vi "图片处理2.vi"() -> ()   [LabVIEW 2018]
uses:
  <vilib>/userdefined/High Color/IMAQdx.ctl
  <vilib>/vision/NI_Vision_Development_Module.lvlib
  <vilib>/vision/driver/NI_Vision_Acquisition_Software.lvlib
panel:
  out "Image 2":T1(plugin-control)
  out "Image":T1(plugin-control)
  in  "File Path":path
  in  "停止":bool
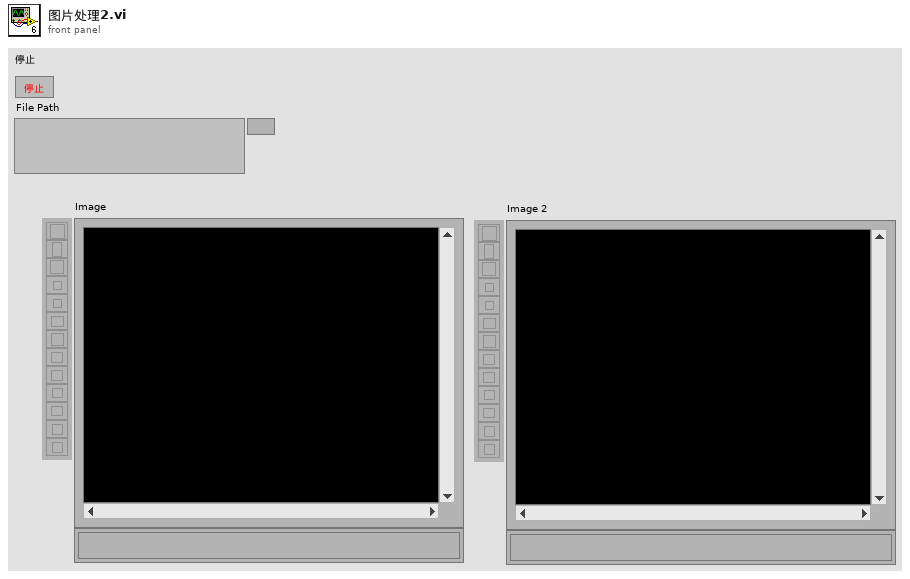
[diagram p1: front panel]
types:
  T1 = typedef "IMAQ Image.ctl" = refnum<image>
  T2 = typedef "IMAQdx.ctl" = refnum<k21>
  T3 = cluster{"Position":cluster{"x":sgl, "y":sgl}, "Angle":sgl, "Scale":sgl, "Score":sgl, "Bounding Box":cluster{"x":sgl, "y":sgl}[]}[]
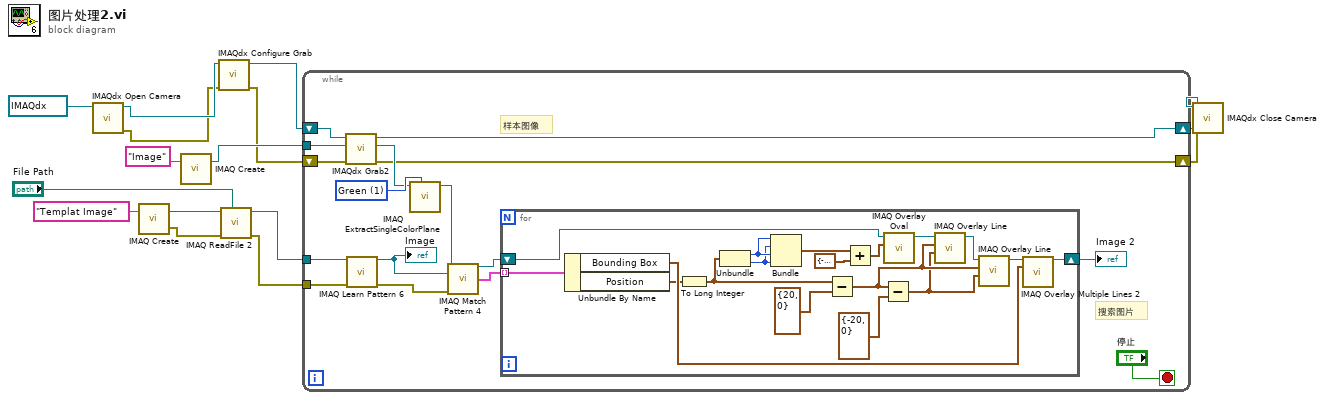
[diagram p0: block diagram]
diagram:
  n1 = call <vilib>:"IMAQdx Open Camera.vi"("Session In"=T2 "cam0") -> ("error out"=w3:errorcluster, "Session Out"=w4:T2)  [unwired: 9 in]
  n2 = call "IMAQ Create"("Image Name"="Templat Image") -> ("New Image"=w15:T1, "error out"=w13:errorcluster)  [unwired: 4 in]
  n3 = call "IMAQ Create"("Image Name"="Image") -> ("New Image"=w10:T1)  [unwired: 4 in, 1 out]
  n4 = call <vilib>:"IMAQdx Configure Grab.vi"("error in"=w3, "Session In"=w4) -> ("error out"=w1:errorcluster, "Session Out"=w2:T2)  [unwired: 8 in]
  n5 = call "IMAQ ReadFile 2"("File Path"="File Path", "error in (no error)"=w13, "Image"=w15) -> ("error out"=w12:errorcluster, "Image Out"=w14:T1)  [unwired: 4 in, 3 out]
  n6 = while {
    tunnel: w14 -> [w31]
    tunnel: w12 -> [w30]
    shift-right: [w17] -> w6
    shift-left: w2 -> [w19]
    shift-right: [w16] -> w5
    shift-left: w1 -> [w18]
    tunnel: w10 -> [w21]
    stop <- "停止" stop-if-true
    w27 = 1 items=["Red", "Green", "Blue", "Hue", "Saturation", "Luminance", "Value", "Intensity"] ("Color Plane")
    # "搜索图片"
    # "样本图像"
    n7 = call <vilib>:"IMAQdx Grab2.vi"("error in"=w18, "Image In"=w21, "Session In"=w19) -> ("error out"=w16:errorcluster, "Image Out"=w20:T1, "Session Out"=w17:T2)  [unwired: 5 in, 1 out]
    n8 = call "IMAQ Learn Pattern 6"("Image"=w31, "error in (no error)"=w30) -> ("Template Image Out"=w24:T1, "error out"=w29:errorcluster)  [unwired: 11 in, 1 out]
    "Image" <- w24
    n9 = call "IMAQ ExtractSingleColorPlane"("Color Plane"=w27, "Image Src"=w20) -> ("Image Dst Out"=w28:T1)  [unwired: 8 in, 1 out]
    n10 = call "IMAQ Match Pattern 4"("Image"=w28, "Template Image"=w24, "error in (no error)"=w29) -> ("Image (duplicate)"=w22:T1, "Matches (real-world)"=w26:T3)  [unwired: 8 in, 3 out]
    n11 = for {
      tunnel: w26 -> [w49] mode=indexing
      shift-right: [w47] -> w23
      shift-left: w22 -> [w42]
      n12 = Unbundle By Name(w49) -> ("Bounding Box"=w48:cluster{"x":sgl, "y":sgl}[], "Position"=w37:cluster{"x":sgl, "y":sgl})
      n13 = To Long Integer(number=w37) -> (32bit integer=w36:cluster{"x":i32, "y":i32})
      n14 = Unbundle(w36) -> ("x"=w46:i32, "y"=w45:i32)
      n15 = Bundle("x"=w46, "y"=w45, "x"=w46, "y"=w45) -> (w44:cluster{"x":i32, "y":i32, "x":i32, "y":i32})  [unwired: 1 in]
      n16 = Subtract(x=w36, y=cluster{"x":i32, "y":i32} {"x"=20, "y"=0}) -> (x-y=w34:cluster{"x":i32, "y":i32})
      n17 = Add(x=w44, y=cluster{"x":i32, "y":i32, "x":i32, "y":i32} {"x"=-10, "y"=-10, "x"=10, "y"=10}) -> (x+y=w41:cluster{"x":i32, "y":i32, "x":i32, "y":i32})
      n18 = Subtract(x=w34, y=cluster{"x":i32, "y":i32} {"x"=-20, "y"=0}) -> (x-y=w32:cluster{"x":i32, "y":i32})
      n19 = call "IMAQ Overlay Oval"("Bounding Rectangle"=w41, "Image"=w42) -> ("Image Out"=w40:T1)  [unwired: 8 in, 1 out]
      n20 = call "IMAQ Overlay Line"("End Point"=w32, "Start Point"=w34, "Image"=w40) -> ("Image Out"=w39:T1)  [unwired: 7 in, 1 out]
      n21 = call "IMAQ Overlay Line"("End Point"=w32, "Start Point"=w34, "Image"=w39) -> ("Image Out"=w38:T1)  [unwired: 7 in, 1 out]
      n22 = call "IMAQ Overlay Multiple Lines 2"("Image"=w38, "Line End Points"=w48) -> ("Image Out"=w47:T1)  [unwired: 12 in, 1 out]
    }
    "Image 2" <- w23
  }
  n23 = call <vilib>:"IMAQdx Close Camera.vi"("error in"=w5, "Session In"=w6) -> ()  [unwired: 9 in, 1 out]
